vi "PQreset.vi"(8 "error in (no error)":errorcluster, 11 "conn":u32) -> (0 "error out":errorcluster, 3 "conn_out":u32)   [LabVIEW 2019, in "libpqlv.lvlib"]
doc: "Resets the communication channel to the server.\n\nThis function will close the connection to the server and attempt to reestablish a new connection to the same server, using all the same parameters previously used. This may be useful for error recovery if a working connection is lost."
uses:
  libpqlv.lvlib
  libpq.dll
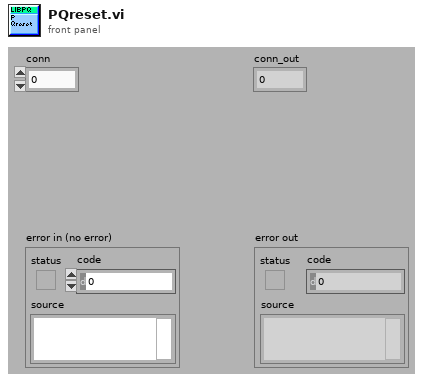
[diagram p1: front panel]
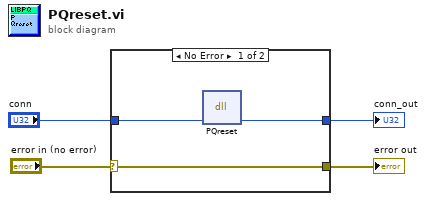
[diagram p0: block diagram]
diagram:
  n1 = case shown="No Error" "error in (no error)" {
    selector: "error in (no error)" -> [w7 w9]
    tunnel: [w7 w9] -> w3
    tunnel: "conn" -> [w6 w8]
    tunnel: [w5 w8] -> w1
    frame No Error {
      n2 = dll-call lib="libpq.*" fn="PQreset"("conn"=w6) -> ("conn"=w5:u32)  [unwired: 4 in, 2 out]
    }
    frame Error {
    }
  }
  "error out" <- w3
  "conn_out" <- w1
